vi "Configure Pulse.vi"(0 "VISA resource name":refnum<visa-resource-name>, 1 "Polarity (0: Normal)":i32(ring) items=["Normal", "Inverted"], 5 "Output Mode (0: Off)":i32(ring) items=["Off", "Pulse Generator", "Gate", "Alarm"], 7 "Pulse Period (1e-7)":dbl=1e-07 min=2e-08 max=2.0 step=1e-08, 9 "Pulse Width (5e-8)":dbl=5e-08 min=1e-08 max=2.0 step=1e-08, 11 "error in (no error)":errorcluster) -> (4 "VISA resource name out":refnum<visa-resource-name>, 15 "error out":errorcluster)   [LabVIEW 2019, in "Pendulum CNT90.lvlib"]
doc: "Controls the rear panel pulse output configuration.\n\n<B>Note:</B> VI is intended for use with CNT-91 only."
uses:
  Pendulum CNT90.lvlib
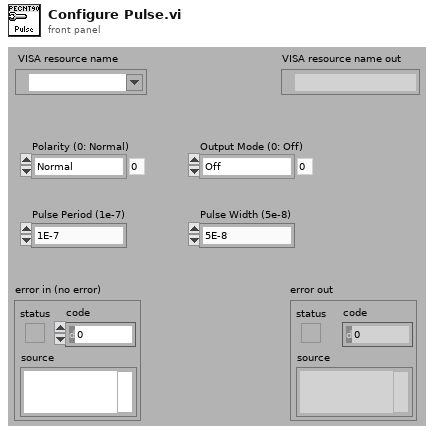
[diagram p1: front panel]
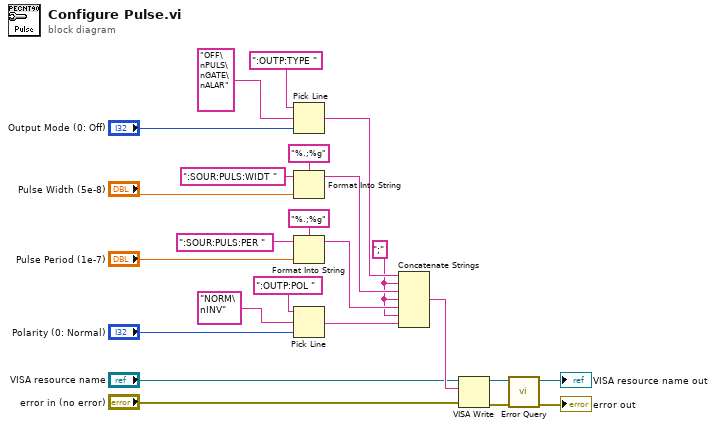
[diagram p0: block diagram]
diagram:
  w12 = ";"
  n1 = Pick Line(string ("")=":OUTP:TYPE ", multi-line string="OFF\nPULS\nGATE\nALAR", line index="Output Mode (0: Off)") -> (output string=w16:string)
  n2 = Format Into String(format string="%.;%g", initial string=":SOUR:PULS:WIDT ", "Pulse Width (5e-8)") -> (resulting string=w15:string)  [unwired: 1 in, 1 out]
  n3 = Format Into String(format string="%.;%g", initial string=":SOUR:PULS:PER ", "Pulse Period (1e-7)") -> (resulting string=w14:string)  [unwired: 1 in, 1 out]
  n4 = Pick Line(string ("")=":OUTP:POL ", multi-line string="NORM\nINV", line index="Polarity (0: Normal)") -> (output string=w13:string)
  n5 = Concatenate Strings(w16, w12, w15, w12, w14, w12, w13) -> (w11:string)
  n6 = VISA Write(VISA resource name="VISA resource name", write buffer=w11, error in (no error)="error in (no error)") -> (VISA resource name out=w3:refnum<visa-resource-name>, error out=w4:errorcluster)  [unwired: 1 out]
  n7 = call "Error Query.vi"("error in (no error)"=w4, "VISA resource name"=w3) -> ("error out"=→"error out":errorcluster, "VISA resource name out"=→"VISA resource name out":refnum<visa-resource-name>)  [unwired: 6 in, 2 out]
